vi "Write unique Name.vi"(8 "error in (no error)":errorcluster, 10 "unique Name":string, 11 "Export in":refnum<class "Export.lvclass">) -> (0 "error out":errorcluster, 3 "Export out":refnum<class "Export.lvclass">)   [LabVIEW 2017, in "CL_G3_VIComponentBuilder.lvlib" / "Export.lvclass"]
uses:
  Export.lvclass
  Export.lvclass/Export.ctl
  Read Export Build Specification.vi
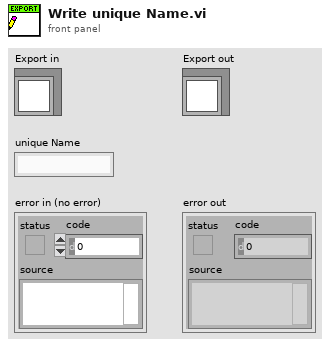
[diagram p1: front panel]
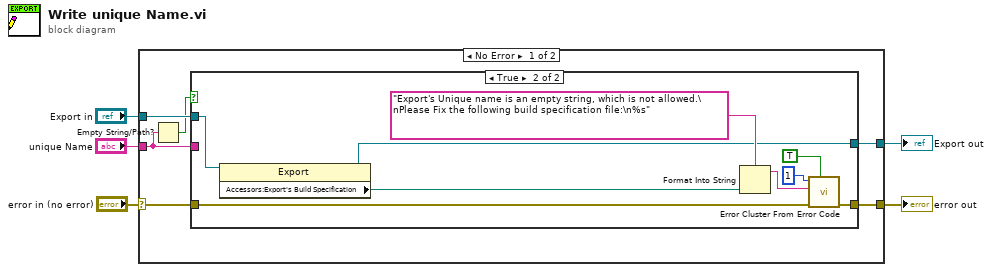
[diagram p0: block diagram]
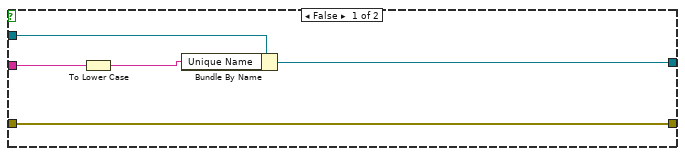
[diagram p2: hidden frame]
diagram:
  n1 = case shown="No Error" "error in (no error)" {
    selector: "error in (no error)" -> [w8 w26]
    tunnel: [w9 w26] -> w4
    tunnel: [w10 w27] -> w2
    tunnel: "Export in" -> [w11 w27]
    tunnel: "unique Name" -> [w6 _]
    frame No Error {
      n2 = Empty String/Path?(string/path=w6) -> (empty?=w7:bool)
      n3 = case shown="True" w7 {
        tunnel: w8 -> [w16 w25]
        tunnel: [w16 w17] -> w9
        tunnel: [w15 w21] -> w10
        tunnel: w6 -> [w14 _]
        tunnel: w11 -> [w12 w18]
        frame False {
          n4 = To Lower Case(string=w14) -> (all lower case string=w13:string)
          n5 = Bundle By Name(cluster=w12, "Unique Name"=w13) -> (w15:refnum<class "Export.lvclass">)
        }
        frame True {
          n6 = property class="Export"(reference=w18) -> (reference out=w21:refnum<class "Export.lvclass">, "Accessors:Export's Build Specification"=w20:path)  [unwired: 1 in, 1 out]
          n7 = Format Into String(format string="Export's Unique name is an empty string, which is not allowed.\nPlease Fix the following build specification file:\n%s" ("error message (\"\")"), w20) -> (resulting string=w19:string)  [unwired: 2 in, 1 out]
          n8 = call <vilib>:"Error Cluster From Error Code.vi"("show call chain? (False)"=TRUE, "error in (no error)"=w25, "error message (\"\")"=w19, "error code (0)"=1) -> ("error out"=w17:errorcluster)  [unwired: 5 in]
        }
      }
    }
    frame Error {
    }
  }
  "error out" <- w4
  "Export out" <- w2
